vi "init Tests.vi"(8 "error in (no error)":errorcluster caption="Fehler (Eingang, kein Fehler)", 11 "CEG4500 Eingang":refnum<class "CEG4500.lvclass"> caption="DNL_LabVIEW Object in") -> (0 "error out":errorcluster caption="Fehler (Ausgang)", 3 "CEG4500 Ausgang":refnum<class "CEG4500.lvclass"> caption="DNL_LabVIEW Object out")   [LabVIEW 2013, in "CEG4500.lvclass"]
uses:
  CEG4500.lvclass
  Tests/Spannungseinbruch/Spannungseinbruch.lvclass
  Tests/Surge/Surge.lvclass
  Tests/Burst/Burst.lvclass
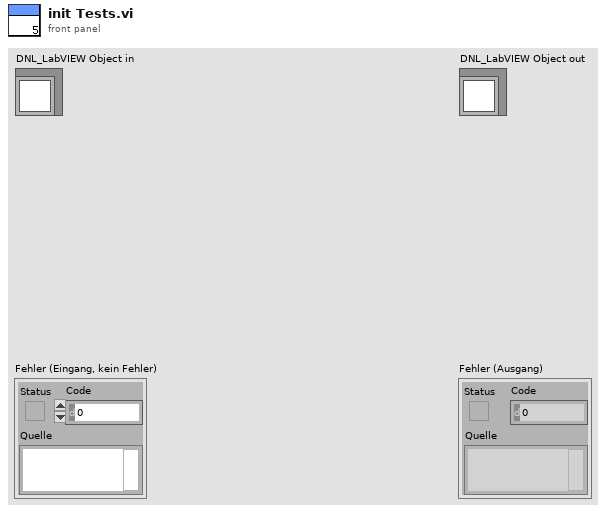
[diagram p1: front panel]
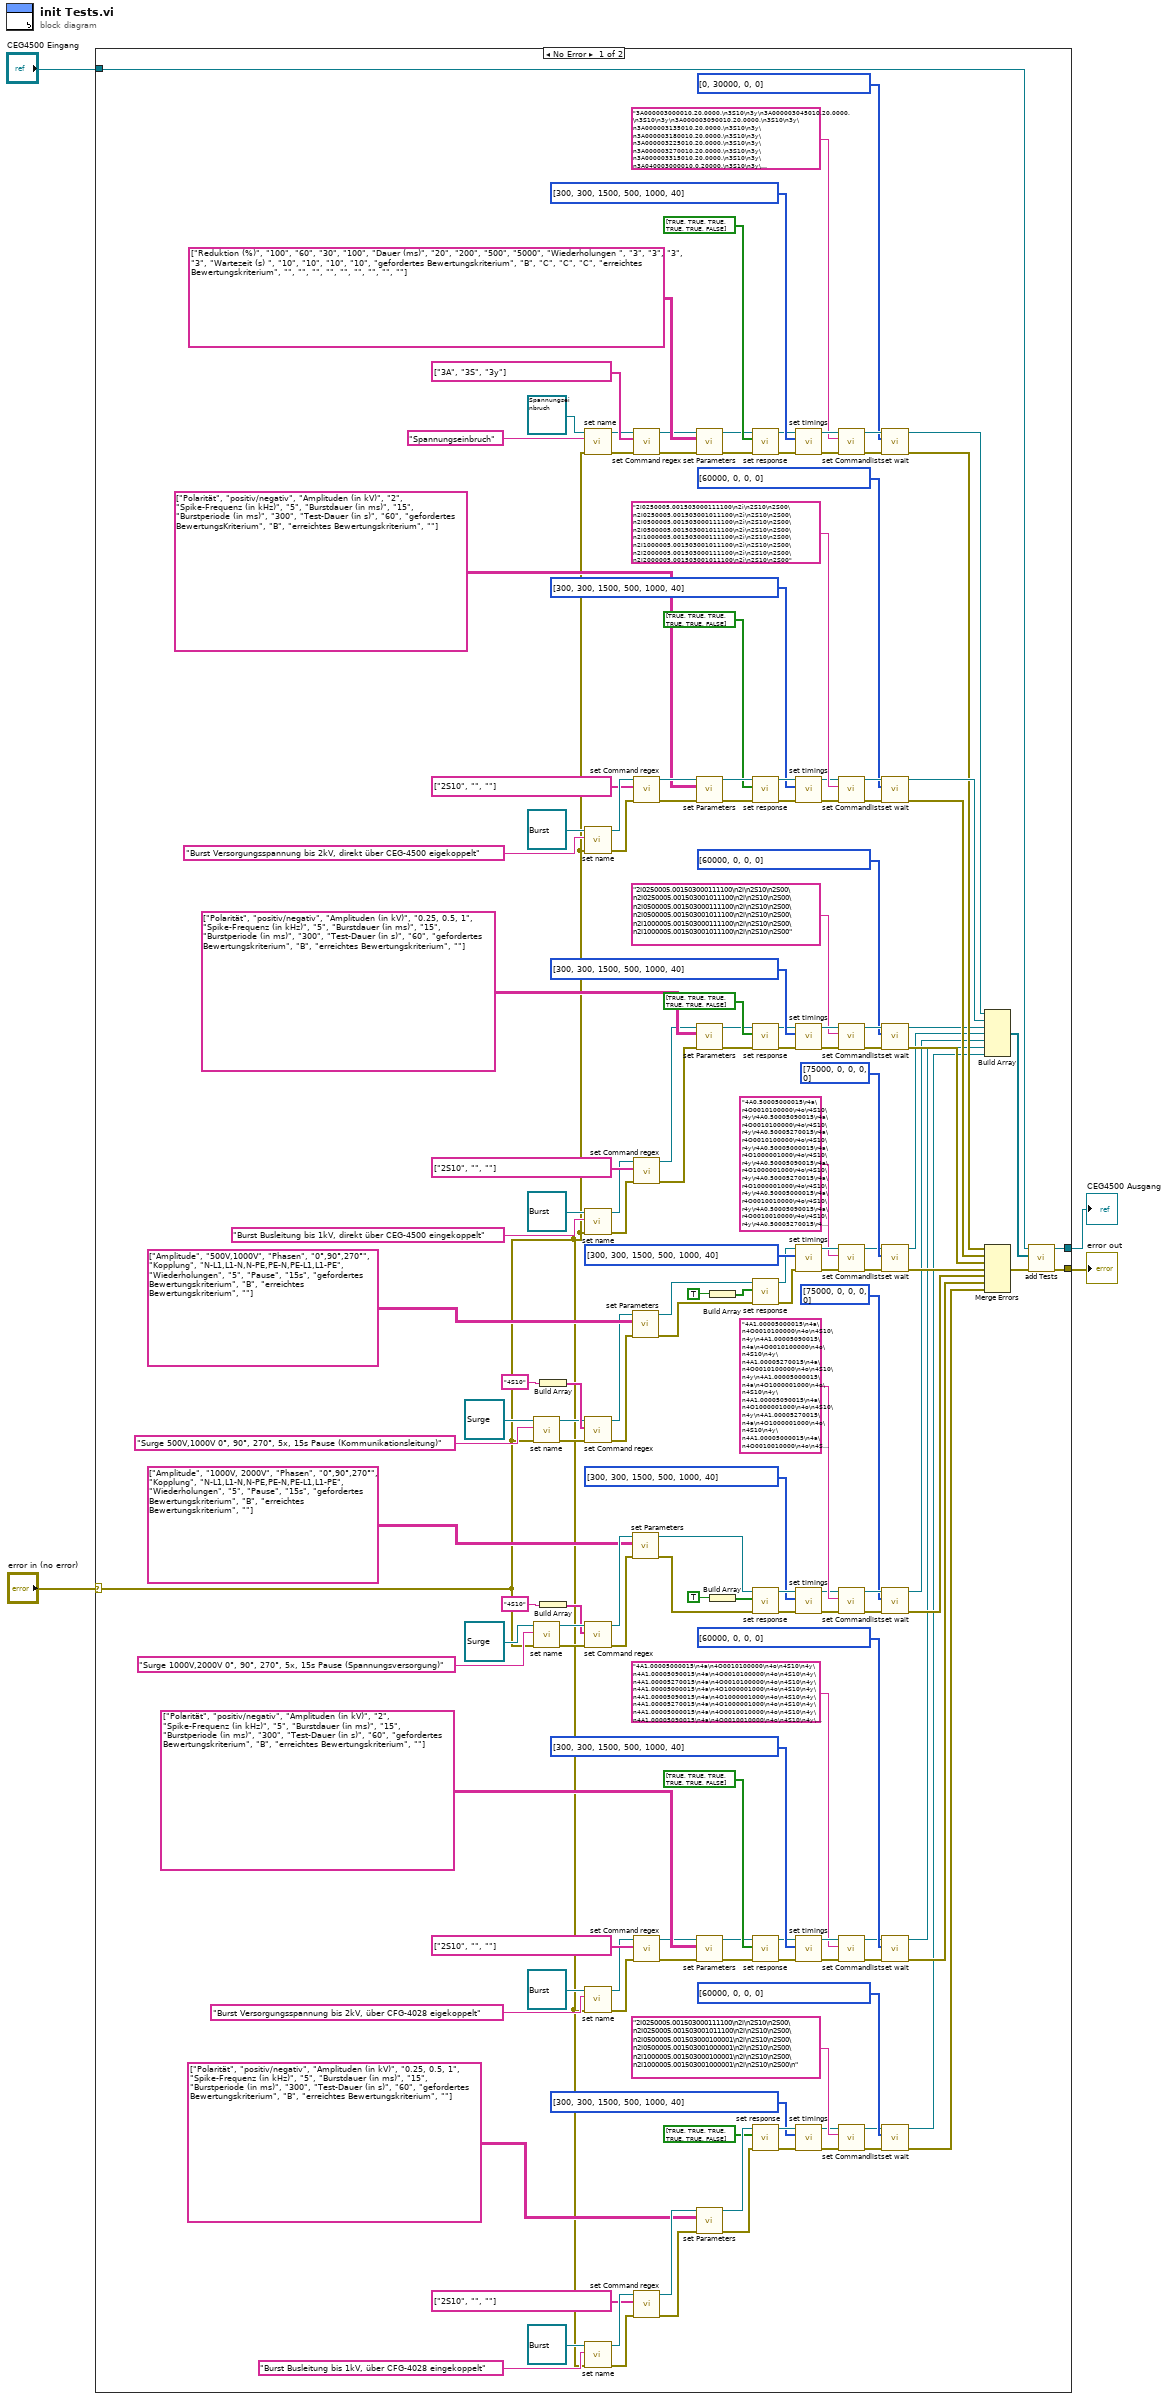
[diagram p0: block diagram]
diagram:
  n1 = case shown="No Error" "error in (no error)" {
    selector: "error in (no error)" -> [w9 w169]
    tunnel: [w167 w169] -> w1
    tunnel: "CEG4500 Eingang" -> [w166 w170]
    tunnel: [w165 w170] -> w3
    frame No Error {
      n2 = call-dynamic "set name.vi"("error in (no error)"=w9, "name"="Surge 500V,1000V 0°, 90°, 270°, 5x, 15s Pause (Kommunikationsleitung)", "TestInterface (Eingang)"=refnum<class "Surge.lvclass"> refnum ("Surge.lvclass")) -> ("error out"=w76:errorcluster, "TestInterface (Ausgang)"=w77:refnum<class "Surge.lvclass">)  [unwired: 7 in]
      n3 = call-dynamic "set name.vi"("error in (no error)"=w9, "name"="Surge 1000V,2000V 0°, 90°, 270°, 5x, 15s Pause (Spannungsversorgung)", "TestInterface (Eingang)"=refnum<class "Surge.lvclass"> refnum ("Surge.lvclass")) -> ("error out"=w73:errorcluster, "TestInterface (Ausgang)"=w72:refnum<class "Surge.lvclass">)  [unwired: 7 in]
      n4 = Build Array("4S10") -> (w82:string[])
      n5 = Build Array("4S10") -> (w67:string[])
      n6 = call-dynamic "set name.vi"("error in (no error)"=w9, "name"="Spannungseinbruch", "TestInterface (Eingang)"=refnum<class "Spannungseinbruch.lvclass"> refnum ("Spannungseinbruch.lvclass")) -> ("error out"=w154:errorcluster, "TestInterface (Ausgang)"=w156:refnum<class "Spannungseinbruch.lvclass">)  [unwired: 7 in]
      n7 = call-dynamic "set name.vi"("error in (no error)"=w9, "name"="Burst Versorgungsspannung bis 2kV, direkt über CEG-4500 eigekoppelt", "TestInterface (Eingang)"=refnum<class "Burst.lvclass"> refnum ("Burst.lvclass")) -> ("error out"=w136:errorcluster, "TestInterface (Ausgang)"=w134:refnum<class "Burst.lvclass">)  [unwired: 7 in]
      n8 = call-dynamic "set name.vi"("error in (no error)"=w9, "name"="Burst Busleitung bis 1kV, direkt über CEG-4500 eingekoppelt", "TestInterface (Eingang)"=refnum<class "Burst.lvclass"> refnum ("Burst.lvclass")) -> ("error out"=w108:errorcluster, "TestInterface (Ausgang)"=w110:refnum<class "Burst.lvclass">)  [unwired: 7 in]
      n9 = call-dynamic "set Command regex.vi"("error in (no error)"=w76, "Command regex"=w82, "TestInterface (Eingang)"=w77) -> ("error out"=w91:errorcluster, "TestInterface (Ausgang)"=w84:refnum<class "Surge.lvclass">)  [unwired: 7 in]
      n10 = call-dynamic "set Command regex.vi"("error in (no error)"=w73, "Command regex"=w67, "TestInterface (Eingang)"=w72) -> ("error out"=w58:errorcluster, "TestInterface (Ausgang)"=w65:refnum<class "Surge.lvclass">)  [unwired: 7 in]
      n11 = call-dynamic "set name.vi"("error in (no error)"=w9, "name"="Burst Versorgungsspannung bis 2kV, über CFG-4028 eigekoppelt", "TestInterface (Eingang)"=refnum<class "Burst.lvclass"> refnum ("Burst.lvclass")) -> ("error out"=w17:errorcluster, "TestInterface (Ausgang)"=w19:refnum<class "Burst.lvclass">)  [unwired: 7 in]
      n12 = call-dynamic "set name.vi"("error in (no error)"=w9, "name"="Burst Busleitung bis 1kV, über CFG-4028 eingekoppelt", "TestInterface (Eingang)"=refnum<class "Burst.lvclass"> refnum ("Burst.lvclass")) -> ("error out"=w41:errorcluster, "TestInterface (Ausgang)"=w39:refnum<class "Burst.lvclass">)  [unwired: 7 in]
      n13 = call-dynamic "set Parameters.vi"("error in (no error)"=w91, "parameters"=string[][] [["Amplitude", "500V,1000V"], ["Phasen", "0°,90°,270°"], ["Kopplung", "N-L1,L1-N,N-PE,PE-N,PE-L1,L1-PE"], ["Wiederholungen", "5"], ["Pause", "15s"], ["gefordertes Bewertungskriterium", "B"], ["erreichtes Bewertungskriterium", ""]], "TestInterface (Eingang)"=w84) -> ("error out"=w92:errorcluster, "TestInterface (Ausgang)"=w89:refnum<class "Surge.lvclass">)  [unwired: 7 in]
      n14 = call-dynamic "set Parameters.vi"("error in (no error)"=w58, "parameters"=string[][] [["Amplitude", "1000V, 2000V"], ["Phasen", "0°,90°,270°"], ["Kopplung", "N-L1,L1-N,N-PE,PE-N,PE-L1,L1-PE"], ["Wiederholungen", "5"], ["Pause", "15s"], ["gefordertes Bewertungskriterium", "B"], ["erreichtes Bewertungskriterium", ""]], "TestInterface (Eingang)"=w65) -> ("error out"=w57:errorcluster, "TestInterface (Ausgang)"=w60:refnum<class "Surge.lvclass">)  [unwired: 7 in]
      n15 = call-dynamic "set Command regex.vi"("error in (no error)"=w154, "Command regex"=string[] ["3A", "3S", "3y"], "TestInterface (Eingang)"=w156) -> ("error out"=w153:errorcluster, "TestInterface (Ausgang)"=w157:refnum<class "Spannungseinbruch.lvclass">)  [unwired: 7 in]
      n16 = call-dynamic "set Command regex.vi"("error in (no error)"=w136, "Command regex"=string[] ["2S10", "", ""], "TestInterface (Eingang)"=w134) -> ("error out"=w137:errorcluster, "TestInterface (Ausgang)"=w133:refnum<class "Burst.lvclass">)  [unwired: 7 in]
      n17 = call-dynamic "set Command regex.vi"("error in (no error)"=w108, "Command regex"=string[] ["2S10", "", ""], "TestInterface (Eingang)"=w110) -> ("error out"=w107:errorcluster, "TestInterface (Ausgang)"=w111:refnum<class "Burst.lvclass">)  [unwired: 7 in]
      n18 = call-dynamic "set Command regex.vi"("error in (no error)"=w17, "Command regex"=string[] ["2S10", "", ""], "TestInterface (Eingang)"=w19) -> ("error out"=w16:errorcluster, "TestInterface (Ausgang)"=w20:refnum<class "Burst.lvclass">)  [unwired: 7 in]
      n19 = call-dynamic "set Command regex.vi"("error in (no error)"=w41, "Command regex"=string[] ["2S10", "", ""], "TestInterface (Eingang)"=w39) -> ("error out"=w42:errorcluster, "TestInterface (Ausgang)"=w38:refnum<class "Burst.lvclass">)  [unwired: 7 in]
      n20 = call-dynamic "set Parameters.vi"("error in (no error)"=w153, "parameters"=string[][] [["Reduktion (%)", "100", "60", "30", "100"], ["Dauer (ms)", "20", "200", "500", "5000"], ["Wiederholungen ", "3", "3", "3", "3"], ["Wartezeit (s) ", "10", "10", "10", "10"], ["gefordertes Bewertungskriterium", "B", "C", "C", "C"], ["erreichtes Bewertungskriterium", "", "", "", ""], ["", "", "", "", ""]], "TestInterface (Eingang)"=w157) -> ("error out"=w152:errorcluster, "TestInterface (Ausgang)"=w158:refnum<class "Spannungseinbruch.lvclass">)  [unwired: 7 in]
      n21 = call-dynamic "set Parameters.vi"("error in (no error)"=w137, "parameters"=string[][] [["Polarität", "positiv/negativ"], ["Amplituden (in kV)", "2"], ["Spike-Frequenz (in kHz)", "5"], ["Burstdauer (in ms)", "15"], ["Burstperiode (in ms)", "300"], ["Test-Dauer (in s)", "60"], ["gefordertes BewertungsKriterium", "B"], ["erreichtes Bewertungskriterium", ""]], "TestInterface (Eingang)"=w133) -> ("error out"=w138:errorcluster, "TestInterface (Ausgang)"=w132:refnum<class "Burst.lvclass">)  [unwired: 7 in]
      n22 = call-dynamic "set Parameters.vi"("error in (no error)"=w107, "parameters"=string[][] [["Polarität", "positiv/negativ"], ["Amplituden (in kV)", "0.25, 0.5, 1"], ["Spike-Frequenz (in kHz)", "5"], ["Burstdauer (in ms)", "15"], ["Burstperiode (in ms)", "300"], ["Test-Dauer (in s)", "60"], ["gefordertes Bewertungskriterium", "B"], ["erreichtes Bewertungskriterium", ""]], "TestInterface (Eingang)"=w111) -> ("error out"=w106:errorcluster, "TestInterface (Ausgang)"=w112:refnum<class "Burst.lvclass">)  [unwired: 7 in]
      n23 = call-dynamic "set Parameters.vi"("error in (no error)"=w16, "parameters"=string[][] [["Polarität", "positiv/negativ"], ["Amplituden (in kV)", "2"], ["Spike-Frequenz (in kHz)", "5"], ["Burstdauer (in ms)", "15"], ["Burstperiode (in ms)", "300"], ["Test-Dauer (in s)", "60"], ["gefordertes Bewertungskriterium", "B"], ["erreichtes Bewertungskriterium", ""]], "TestInterface (Eingang)"=w20) -> ("error out"=w15:errorcluster, "TestInterface (Ausgang)"=w21:refnum<class "Burst.lvclass">)  [unwired: 7 in]
      n24 = call-dynamic "set Parameters.vi"("error in (no error)"=w42, "parameters"=string[][] [["Polarität", "positiv/negativ"], ["Amplituden (in kV)", "0.25, 0.5, 1"], ["Spike-Frequenz (in kHz)", "5"], ["Burstdauer (in ms)", "15"], ["Burstperiode (in ms)", "300"], ["Test-Dauer (in s)", "60"], ["gefordertes Bewertungskriterium", "B"], ["erreichtes Bewertungskriterium", ""]], "TestInterface (Eingang)"=w38) -> ("error out"=w43:errorcluster, "TestInterface (Ausgang)"=w37:refnum<class "Burst.lvclass">)  [unwired: 7 in]
      n25 = Build Array(TRUE) -> (w85:bool[])
      n26 = Build Array(TRUE) -> (w64:bool[])
      n27 = call-dynamic "set response.vi"("error in (no error)"=w152, "response?"=bool[] [TRUE, TRUE, TRUE, TRUE, TRUE, FALSE], "TestInterface (Eingang)"=w158) -> ("error out"=w151:errorcluster, "TestInterface (Ausgang)"=w159:refnum<class "Spannungseinbruch.lvclass">)  [unwired: 7 in]
      n28 = call-dynamic "set response.vi"("error in (no error)"=w138, "response?"=bool[] [TRUE, TRUE, TRUE, TRUE, TRUE, FALSE], "TestInterface (Eingang)"=w132) -> ("error out"=w139:errorcluster, "TestInterface (Ausgang)"=w131:refnum<class "Burst.lvclass">)  [unwired: 7 in]
      n29 = call-dynamic "set response.vi"("error in (no error)"=w106, "response?"=bool[] [TRUE, TRUE, TRUE, TRUE, TRUE, FALSE], "TestInterface (Eingang)"=w112) -> ("error out"=w105:errorcluster, "TestInterface (Ausgang)"=w113:refnum<class "Burst.lvclass">)  [unwired: 7 in]
      n30 = call-dynamic "set response.vi"("error in (no error)"=w92, "response?"=w85, "TestInterface (Eingang)"=w89) -> ("error out"=w93:errorcluster, "TestInterface (Ausgang)"=w88:refnum<class "Surge.lvclass">)  [unwired: 7 in]
      n31 = call-dynamic "set response.vi"("error in (no error)"=w57, "response?"=w64, "TestInterface (Eingang)"=w60) -> ("error out"=w56:errorcluster, "TestInterface (Ausgang)"=w61:refnum<class "Surge.lvclass">)  [unwired: 7 in]
      n32 = call-dynamic "set response.vi"("error in (no error)"=w15, "response?"=bool[] [TRUE, TRUE, TRUE, TRUE, TRUE, FALSE], "TestInterface (Eingang)"=w21) -> ("error out"=w14:errorcluster, "TestInterface (Ausgang)"=w22:refnum<class "Burst.lvclass">)  [unwired: 7 in]
      n33 = call-dynamic "set response.vi"("error in (no error)"=w43, "response?"=bool[] [TRUE, TRUE, TRUE, TRUE, TRUE, FALSE], "TestInterface (Eingang)"=w37) -> ("error out"=w44:errorcluster, "TestInterface (Ausgang)"=w36:refnum<class "Burst.lvclass">)  [unwired: 7 in]
      n34 = call-dynamic "set timings.vi"("error in (no error)"=w151, "timings"=i32[] [300, 300, 1500, 500, 1000, 40] ("Timings"), "TestInterface (Eingang)"=w159) -> ("error out"=w150:errorcluster, "TestInterface (Ausgang)"=w155:refnum<class "Spannungseinbruch.lvclass">)  [unwired: 7 in]
      n35 = call-dynamic "set timings.vi"("error in (no error)"=w139, "timings"=i32[] [300, 300, 1500, 500, 1000, 40] ("Timings"), "TestInterface (Eingang)"=w131) -> ("error out"=w140:errorcluster, "TestInterface (Ausgang)"=w135:refnum<class "Burst.lvclass">)  [unwired: 7 in]
      n36 = call-dynamic "set timings.vi"("error in (no error)"=w105, "timings"=i32[] [300, 300, 1500, 500, 1000, 40] ("Timings"), "TestInterface (Eingang)"=w113) -> ("error out"=w104:errorcluster, "TestInterface (Ausgang)"=w109:refnum<class "Burst.lvclass">)  [unwired: 7 in]
      n37 = call-dynamic "set timings.vi"("error in (no error)"=w93, "timings"=u32[] [300, 300, 1500, 500, 1000, 40] ("timeout"), "TestInterface (Eingang)"=w88) -> ("error out"=w94:errorcluster, "TestInterface (Ausgang)"=w87:refnum<class "Surge.lvclass">)  [unwired: 7 in]
      n38 = call-dynamic "set timings.vi"("error in (no error)"=w56, "timings"=u32[] [300, 300, 1500, 500, 1000, 40] ("timeout"), "TestInterface (Eingang)"=w61) -> ("error out"=w55:errorcluster, "TestInterface (Ausgang)"=w62:refnum<class "Surge.lvclass">)  [unwired: 7 in]
      n39 = call-dynamic "set timings.vi"("error in (no error)"=w14, "timings"=i32[] [300, 300, 1500, 500, 1000, 40] ("Timings"), "TestInterface (Eingang)"=w22) -> ("error out"=w13:errorcluster, "TestInterface (Ausgang)"=w18:refnum<class "Burst.lvclass">)  [unwired: 7 in]
      n40 = call-dynamic "set timings.vi"("error in (no error)"=w44, "timings"=i32[] [300, 300, 1500, 500, 1000, 40] ("Timings"), "TestInterface (Eingang)"=w36) -> ("error out"=w45:errorcluster, "TestInterface (Ausgang)"=w40:refnum<class "Burst.lvclass">)  [unwired: 7 in]
      n41 = call-dynamic "set Commandlist.vi"("error in (no error)"=w150, "Commandlist"="3A000003000010.20.0000.\n3S10\n3y\n3A000003045010.20.0000.\n3S10\n3y\n3A000003090010.20.0000.\n3S10\n3y\n3A000003135010.20.0000.\n3S10\n3y\n3A000003180010.20.0000.\n3S10\n3y\n3A000003225010.20.0000.\n3S10\n3y\n3A000003270010.20.0000.\n3S10\n3y\n3A000003315010.20.0000.\n3S10\n3y\n3A040003000010.0.20000.\n3S10\n3y\n3A040003045010.0.20000.\n3S10\n3y\n3A040003090010.0.20000.\n3S10\n3y\n3A040003135010.0.20000.\n3S10\n3y\n3A040003180010.0.20000.\n3S10\n3y\n3A040003225010.0.20000.\n3S10\n3y\n3A040003270010.0.20000.\n3S10\n3y\n3A040003315010.0.20000.\n3S10\n3y\n3A070003000010.0.50000.\n3S10\n3y\n3A070003045010.0.50000.\n3S10\n3y\n3A070003090010.0.50000.\n3S10\n3y\n3A070003135010.0.50000.\n3S10\n3y\n3A070003180010.0.50000.\n3S10\n3y\n3A070003225010.0.50000.\n3S10\n3y\n3A070003270010.0.50000.\n3S10\n3y\n3A070003315010.0.50000.\n3S10\n3y\n3A000003000010.5.00000.\n3S10\n3y\n3y\n", "TestInterface (Eingang)"=w155) -> ("error out"=w148:errorcluster, "TestInterface (Ausgang)"=w147:refnum<class "Spannungseinbruch.lvclass">)  [unwired: 7 in]
      n42 = call-dynamic "set Commandlist.vi"("error in (no error)"=w140, "Commandlist"="2I0250005.001503000111100\n2i\n2S10\n2S00\n2I0250005.001503001011100\n2i\n2S10\n2S00\n2I0500005.001503000111100\n2i\n2S10\n2S00\n2I0500005.001503001011100\n2i\n2S10\n2S00\n2I1000005.001503000111100\n2i\n2S10\n2S00\n2I1000005.001503001011100\n2i\n2S10\n2S00\n2I2000005.001503000111100\n2i\n2S10\n2S00\n2I2000005.001503001011100\n2i\n2S10\n2S00", "TestInterface (Eingang)"=w135) -> ("error out"=w141:errorcluster, "TestInterface (Ausgang)"=w142:refnum<class "Burst.lvclass">)  [unwired: 7 in]
      n43 = call-dynamic "set Commandlist.vi"("error in (no error)"=w104, "Commandlist"="2I0250005.001503000111100\n2i\n2S10\n2S00\n2I0250005.001503001011100\n2i\n2S10\n2S00\n2I0500005.001503000111100\n2i\n2S10\n2S00\n2I0500005.001503001011100\n2i\n2S10\n2S00\n2I1000005.001503000111100\n2i\n2S10\n2S00\n2I1000005.001503001011100\n2i\n2S10\n2S00", "TestInterface (Eingang)"=w109) -> ("error out"=w103:errorcluster, "TestInterface (Ausgang)"=w102:refnum<class "Burst.lvclass">)  [unwired: 7 in]
      n44 = call-dynamic "set Commandlist.vi"("error in (no error)"=w94, "Commandlist"="4A0.50005000015\r4a\r4O0010100000\r4o\r4S10\r4y\r4A0.50005090015\r4a\r4O0010100000\r4o\r4S10\r4y\r4A0.50005270015\r4a\r4O0010100000\r4o\r4S10\r4y\r4A0.50005000015\r4a\r4O1000001000\r4o\r4S10\r4y\r4A0.50005090015\r4a\r4O1000001000\r4o\r4S10\r4y\r4A0.50005270015\r4a\r4O1000001000\r4o\r4S10\r4y\r4A0.50005000015\r4a\r4O0010010000\r4o\r4S10\r4y\r4A0.50005090015\r4a\r4O0010010000\r4o\r4S10\r4y\r4A0.50005270015\r4a\r4O0010010000\r4o\r4S10\r4y\r4A0.50005000015\r4a\r4O0100001000\r4o\r4S10\r4y\r4A0.50005090015\r4a\r4O0100001000\r4o\r4S10\r4y\r4A0.50005270015\r4a\r4O0100001000\r4o\r4S10\r4y\r4A0.50005000015\r4a\r4O0100100000\r4o\r4S10\r4y\r4A0.50005090015\r4a\r4O0100100000\r4o\r4S10\r4y\r4A0.50005270015\r4a\r4O0100100000\r4o\r4S10\r4y\r4A0.50005000015\r4a\r4O1000010000\r4o\r4S10\r4y\r4A0.50005090015\r4a\r4O1000010000\r4o\r4S10\r4y\r4A0.50005270015\r4a\r4O1000010000\r4o\r4S10\r4y\n4A1.00005000015\r4a\r4O0010100000\r4o\r4S10\r4y\r4A1.00005090015\r4a\r4O0010100000\r4o\r4S10\r4y\r4A1.00005270015\r4a\r4O0010100000\r4o\r4S10\r4y\r4A1.00005000015\r4a\r4O1000001000\r4o\r4S10\r4y\r4A1.00005090015\r4a\r4O1000001000\r4o\r4S10\r4y\r4A1.00005270015\r4a\r4O1000001000\r4o\r4S10\r4y\r4A1.00005000015\r4a\r4O0010010000\r4o\r4S10\r4y\r4A1.00005090015\r4a\r4O0010010000\r4o\r4S10\r4y\r4A1.00005270015\r4a\r4O0010010000\r4o\r4S10\r4y\r4A1.00005000015\r4a\r4O0100001000\r4o\r4S10\r4y\r4A1.00005090015\r4a\r4O0100001000\r4o\r4S10\r4y\r4A1.00005270015\r4a\r4O0100001000\r4o\r4S10\r4y\r4A1.00005000015\r4a\r4O0100100000\r4o\r4S10\r4y\r4A1.00005090015\r4a\r4O0100100000\r4o\r4S10\r4y\r4A1.00005270015\r4a\r4O0100100000\r4o\r4S10\r4y\r4A1.00005000015\r4a\r4O1000010000\r4o\r4S10\r4y\r4A1.00005090015\r4a\r4O1000010000\r4o\r4S10\r4y\r4A1.00005270015\r4a\r4O1000010000\r4o\r4S10\r4y\r", "TestInterface (Eingang)"=w87) -> ("error out"=w95:errorcluster, "TestInterface (Ausgang)"=w86:refnum<class "Surge.lvclass">)  [unwired: 7 in]
      n45 = call-dynamic "set Commandlist.vi"("error in (no error)"=w55, "Commandlist"="4A1.00005000015\n4a\n4O0010100000\n4o\n4S10\n4y\n4A1.00005090015\n4a\n4O0010100000\n4o\n4S10\n4y\n4A1.00005270015\n4a\n4O0010100000\n4o\n4S10\n4y\n4A1.00005000015\n4a\n4O1000001000\n4o\n4S10\n4y\n4A1.00005090015\n4a\n4O1000001000\n4o\n4S10\n4y\n4A1.00005270015\n4a\n4O1000001000\n4o\n4S10\n4y\n4A1.00005000015\n4a\n4O0010010000\n4o\n4S10\n4y\n4A1.00005090015\n4a\n4O0010010000\n4o\n4S10\n4y\n4A1.00005270015\n4a\n4O0010010000\n4o\n4S10\n4y\n4A1.00005000015\n4a\n4O0100001000\n4o\n4S10\n4y\n4A1.00005090015\n4a\n4O0100001000\n4o\n4S10\n4y\n4A1.00005270015\n4a\n4O0100001000\n4o\n4S10\n4y\n4A1.00005000015\n4a\n4O0100100000\n4o\n4S10\n4y\n4A1.00005090015\n4a\n4O0100100000\n4o\n4S10\n4y\n4A1.00005270015\n4a\n4O0100100000\n4o\n4S10\n4y\n4A1.00005000015\n4a\n4O1000010000\n4o\n4S10\n4y\n4A1.00005090015\n4a\n4O1000010000\n4o\n4S10\n4y\n4A1.00005270015\n4a\n4O1000010000\n4o\n4S10\n4y\n4A2.00005000015\n4a\n4O0010010000\n4o\n4S10\n4y\n4A2.00005090015\n4a\n4O0010010000\n4o\n4S10\n4y\n4A2.00005270015\n4a\n4O0010010000\n4o\n4S10\n4y\n4A2.00005000015\n4a\n4O0100001000\n4o\n4S10\n4y\n4A2.00005090015\n4a\n4O0100001000\n4o\n4S10\n4y\n4A2.00005270015\n4a\n4O0100001000\n4o\n4S10\n4y\n4A2.00005000015\n4a\n4O0100100000\n4o\n4S10\n4y\n4A2.00005090015\n4a\n4O0100100000\n4o\n4S10\n4y\n4A2.00005270015\n4a\n4O0100100000\n4o\n4S10\n4y\n4A2.00005000015\n4a\n4O1000010000\n4o\n4S10\n4y\n4A2.00005090015\n4a\n4O1000010000\n4o\n4S10\n4y\n4A2.00005270015\n4a\n4O1000010000\n4o\n4S10\n4y", "TestInterface (Eingang)"=w62) -> ("error out"=w54:errorcluster, "TestInterface (Ausgang)"=w63:refnum<class "Surge.lvclass">)  [unwired: 7 in]
      n46 = call-dynamic "set Commandlist.vi"("error in (no error)"=w13, "Commandlist"="4A1.00005000015\n4a\n4O0010100000\n4o\n4S10\n4y\n4A1.00005090015\n4a\n4O0010100000\n4o\n4S10\n4y\n4A1.00005270015\n4a\n4O0010100000\n4o\n4S10\n4y\n4A1.00005000015\n4a\n4O1000001000\n4o\n4S10\n4y\n4A1.00005090015\n4a\n4O1000001000\n4o\n4S10\n4y\n4A1.00005270015\n4a\n4O1000001000\n4o\n4S10\n4y\n4A1.00005000015\n4a\n4O0010010000\n4o\n4S10\n4y\n4A1.00005090015\n4a\n4O0010010000\n4o\n4S10\n4y\n4A1.00005270015\n4a\n4O0010010000\n4o\n4S10\n4y\n4A1.00005000015\n4a\n4O0100001000\n4o\n4S10\n4y\n4A1.00005090015\n4a\n4O0100001000\n4o\n4S10\n4y\n4A1.00005270015\n4a\n4O0100001000\n4o\n4S10\n4y\n4A1.00005000015\n4a\n4O0100100000\n4o\n4S10\n4y\n4A1.00005090015\n4a\n4O0100100000\n4o\n4S10\n4y\n4A1.00005270015\n4a\n4O0100100000\n4o\n4S10\n4y\n4A1.00005000015\n4a\n4O1000010000\n4o\n4S10\n4y\n4A1.00005090015\n4a\n4O1000010000\n4o\n4S10\n4y\n4A1.00005270015\n4a\n4O1000010000\n4o\n4S10\n4y\n4A2.00005000015\n4a\n4O0010010000\n4o\n4S10\n4y\n4A2.00005090015\n4a\n4O0010010000\n4o\n4S10\n4y\n4A2.00005270015\n4a\n4O0010010000\n4o\n4S10\n4y\n4A2.00005000015\n4a\n4O0100001000\n4o\n4S10\n4y\n4A2.00005090015\n4a\n4O0100001000\n4o\n4S10\n4y\n4A2.00005270015\n4a\n4O0100001000\n4o\n4S10\n4y\n4A2.00005000015\n4a\n4O0100100000\n4o\n4S10\n4y\n4A2.00005090015\n4a\n4O0100100000\n4o\n4S10\n4y\n4A2.00005270015\n4a\n4O0100100000\n4o\n4S10\n4y\n4A2.00005000015\n4a\n4O1000010000\n4o\n4S10\n4y\n4A2.00005090015\n4a\n4O1000010000\n4o\n4S10\n4y\n4A2.00005270015\n4a\n4O1000010000\n4o\n4S10\n4y", "TestInterface (Eingang)"=w18) -> ("error out"=w12:errorcluster, "TestInterface (Ausgang)"=w11:refnum<class "Burst.lvclass">)  [unwired: 7 in]
      n47 = call-dynamic "set Commandlist.vi"("error in (no error)"=w45, "Commandlist"="2I0250005.001503000111100\n2i\n2S10\n2S00\n2I0250005.001503001011100\n2i\n2S10\n2S00\n2I0500005.001503000100001\n2i\n2S10\n2S00\n2I0500005.001503001000001\n2i\n2S10\n2S00\n2I1000005.001503000100001\n2i\n2S10\n2S00\n2I1000005.001503001000001\n2i\n2S10\n2S00\n", "TestInterface (Eingang)"=w40) -> ("error out"=w46:errorcluster, "TestInterface (Ausgang)"=w47:refnum<class "Burst.lvclass">)  [unwired: 7 in]
      n48 = call-dynamic "set wait.vi"("error in (no error)"=w148, "wait"=i32[] [0, 30000, 0, 0] ("Timings"), "TestInterface in"=w147) -> ("error out"=w121:errorcluster, "TestInterface out"=w146:refnum<class "Spannungseinbruch.lvclass">)  [unwired: 7 in]
      n49 = call-dynamic "set wait.vi"("error in (no error)"=w141, "wait"=i32[] [60000, 0, 0, 0] ("Timings"), "TestInterface in"=w142) -> ("error out"=w122:errorcluster, "TestInterface out"=w123:refnum<class "Burst.lvclass">)  [unwired: 7 in]
      n50 = call-dynamic "set wait.vi"("error in (no error)"=w103, "wait"=i32[] [60000, 0, 0, 0] ("Timings"), "TestInterface in"=w102) -> ("error out"=w100:errorcluster, "TestInterface out"=w99:refnum<class "Burst.lvclass">)  [unwired: 7 in]
      n51 = call-dynamic "set wait.vi"("error in (no error)"=w95, "wait"=i32[] [75000, 0, 0, 0, 0], "TestInterface in"=w86) -> ("error out"=w75:errorcluster, "TestInterface out"=w74:refnum<class "Surge.lvclass">)  [unwired: 7 in]
      n52 = call-dynamic "set wait.vi"("error in (no error)"=w54, "wait"=i32[] [75000, 0, 0, 0, 0], "TestInterface in"=w63) -> ("error out"=w51:errorcluster, "TestInterface out"=w50:refnum<class "Surge.lvclass">)  [unwired: 7 in]
      n53 = call-dynamic "set wait.vi"("error in (no error)"=w12, "wait"=i32[] [60000, 0, 0, 0] ("Timings"), "TestInterface in"=w11) -> ("error out"=w8:errorcluster, "TestInterface out"=w7:refnum<class "Burst.lvclass">)  [unwired: 7 in]
      n54 = call-dynamic "set wait.vi"("error in (no error)"=w46, "wait"=i32[] [60000, 0, 0, 0] ("Timings"), "TestInterface in"=w47) -> ("error out"=w5:errorcluster, "TestInterface out"=w6:refnum<class "Burst.lvclass">)  [unwired: 7 in]
      n55 = Build Array(w146, w123, w99, w74, w50, w7, w6) -> (w168:refnum<class "TestInterface.lvclass">[])
      n56 = Merge Errors(w121, w122, w100, w75, w51, w8, w5) -> (w120:errorcluster)
      n57 = call-dynamic "add Tests.vi"("error in (no error)"=w120, "Tests"=w168, "DeviceInterface (Eingang)"=w166) -> ("error out"=w167:errorcluster, "DeviceInterface (Ausgang)"=w165:refnum<class "CEG4500.lvclass">)  [unwired: 7 in]
    }
    frame Error {
    }
  }
  "error out" <- w1
  "CEG4500 Ausgang" <- w3
